vi "FGV Auswertung sammeln.vi"(6 "Aktion":T1, 8 "error in (no error)":errorcluster caption="Fehler (Eingang, kein Fehler)", 10 "Auswertung":cluster{sgl[], sgl[], bool[]}, 11 "LINVer Auswertung":string[][](array[string])) -> (0 "error out":errorcluster caption="Fehler (Ausgang)", 2 "Auswertung out":cluster{sgl[], sgl[], bool[]}, 3 "LINVer Auswertung":string[][](array[string]))   [LabVIEW 2020, in "Linearisierung v2.lvlib" / "Linearity verification 1065-307.lvlib"]
uses:
  Linearity verification 1065-307.lvlib
  Aktion FGV Auswertung sammeln.ctl
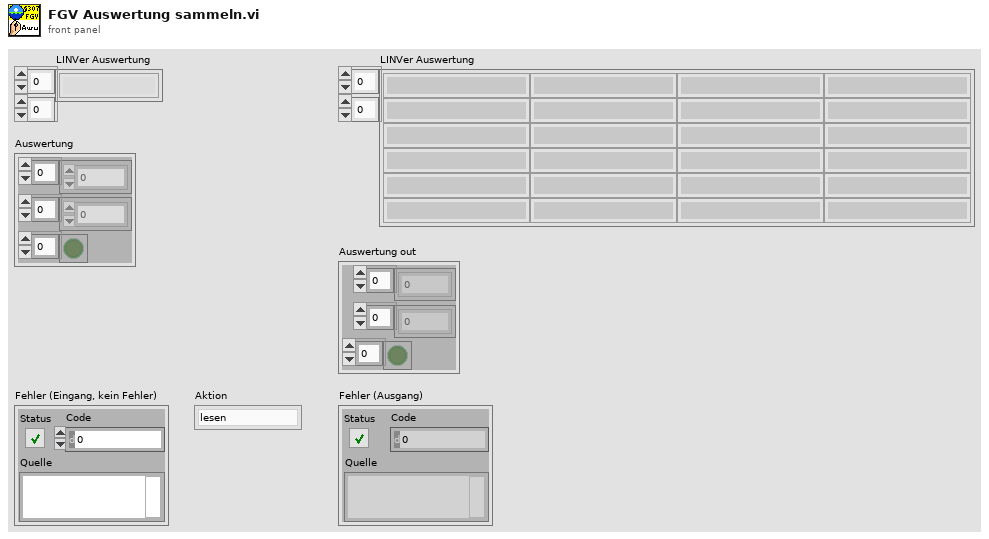
[diagram p1: front panel]
types:
  T1 = typedef "Linearisierung v2.lvlib/Linearity verification 1065-307.lvlib/Aktion FGV Auswertung sammeln.ctl" = enum16{"lesen", "Auswertung", "löschen"}
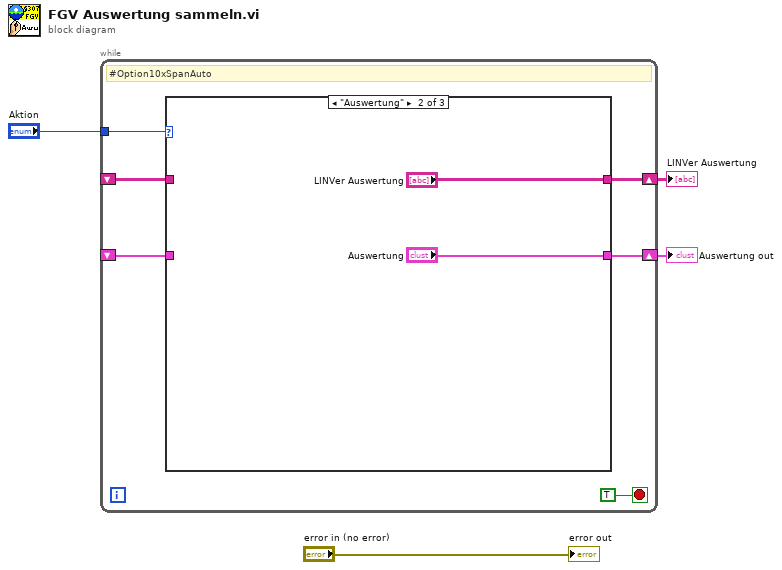
[diagram p0: block diagram]
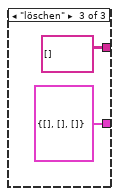
[diagram p3: hidden frame]
diagram:
  n1 = while {
    tunnel: "Aktion" -> [w9]
    shift-right: [w8] -> w3
    shift-left: _ -> [w7]
    shift-right: [w6] -> w2
    shift-left: _ -> [w5]
    stop <- TRUE stop-if-true
    # "#Option10xSpanAuto"
    n2 = case shown="\"Auswertung\"" w9 {
      tunnel: [w12 "LINVer Auswertung" string[][] [] ("LINVer Auswertung")] -> w8
      tunnel: w7 -> [w12 _ _]
      tunnel: [w11 "Auswertung" cluster{sgl[], sgl[], bool[]} {[], [], []} ("Auswertung")] -> w6
      tunnel: w5 -> [w11 _ _]
      frame "lesen", Default {
      }
      frame "Auswertung" {
      }
      frame "löschen" {
      }
    }
  }
  "LINVer Auswertung" <- w3
  "Auswertung out" <- w2
  "error out" <- "error in (no error)"
